vi "Robot Build.vi"() -> ()   [LabVIEW 2011]
uses:
  Controls/Robot Build.ctl
panel:
  in  "Robot Build":T1=enum."Competition Bot"
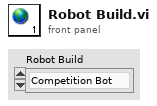
[diagram p1: front panel]
types:
  T1 = typedef "Robot Build.ctl" = enum16{"Practice Bot", "Competition Bot"}
diagram:
